vi "OutputLimeLight.vi"   [LabVIEW 2020]
doc: "This VI sends commands to the LimeLight camera."
uses:
  a4c4c9eb-852e-4134-b059-2c269de838ae.vi
  bed327a2-98d3-4965-916e-7305edcf582b.vi
  9959ab12-4f3e-4c63-8bb4-e3e2fa624083.vi
  a4c4c9eb-852e-4134-b059-2c269de838ae.vi/77c742ae-e671-49bb-a825-a6e8cebc9f63.vi
  bed327a2-98d3-4965-916e-7305edcf582b.vi/77c742ae-e671-49bb-a825-a6e8cebc9f63.vi
  9959ab12-4f3e-4c63-8bb4-e3e2fa624083.vi/77c742ae-e671-49bb-a825-a6e8cebc9f63.vi
  <vilib>/Rock Robotics/Network Tables/NT Read Number.vi
  GlobalMiscellaneous.vi
  GlobalDriverStationData.vi
  <vilib>/Rock Robotics/Network Tables/NT Write Value.vi
  <vilib>/Rock Robotics/Network Tables/NT Write Number.vi
types:
  T1 = enum16{"Side-by-Side", "PiP Main", "PiP Secondary"}
  T2 = enum16{"Boot Up", "Camera Override", "HUB Targeting", "CARGO Tracking"}
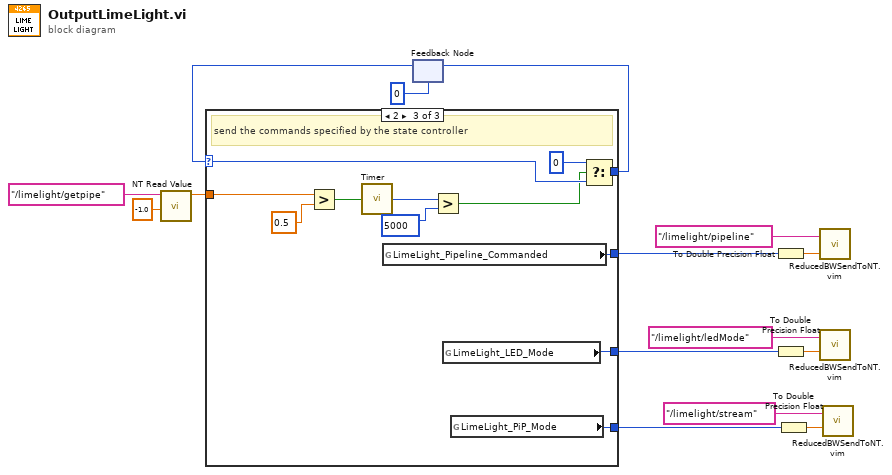
[diagram p0: block diagram]
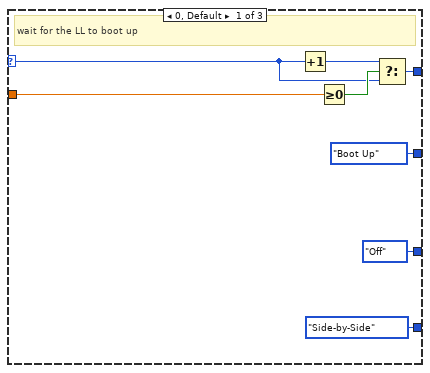
[diagram p2: hidden frame]
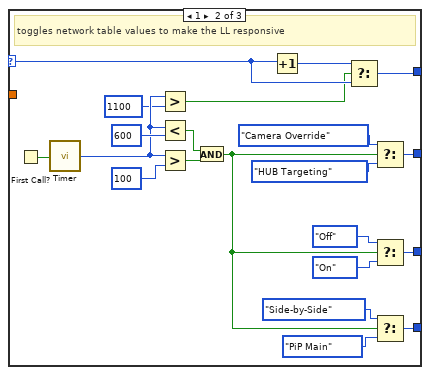
[diagram p3: hidden frame]
diagram:
  n1 = call-poly <vilib>:"NT Read Value.vi"("Default Value"=-1.0, "Name"="/limelight/getpipe") -> ("Numeric"=w6:dbl)  [unwired: 8 in, 1 out]
  n2 = feedback #1(0) -> (w10:i32)
  n3 = case shown="2" w10 {
    selector: w10 -> [w21 w43 w54]
    tunnel: [w20 w42 w55] -> w11
    tunnel: [T2."Boot Up" w28 w46] -> w5
    tunnel: [enum16{"Pipeline Setting", "Off", "Blink", "On"}."Off" ("LimeLight_LED_Mode") w29 w56] -> w4
    tunnel: w6 -> [w17 _ w52]
    tunnel: [T1."Side-by-Side" ("LimeLight_PiP_Mode") w27 w45] -> w1
    frame 0, Default {
      # "wait for the LL to boot up"
      n4 = Increment(x=w21) -> (x+1=w22:i32)
      n5 = Greater Or Equal To 0?(x=w17) -> (x >= 0?=w23:bool)
      n6 = Select(t=w22, s=w23, f=w21) -> (s? t:f=w20:i32)
    }
    frame 1 {
      # "toggles network table values to make the LL responsive"
      n7 = First Call?() -> (First Call?: T/F=w41:bool)
      n8 = call "Timer.vi"("Reset Timer"=w41) -> ("Time (ms)"=w34:u32)
      n9 = Greater?(x=w34, y=u32 1100) -> (0:w32:bool)
      n10 = Less?(x=w34, y=u32 600) -> (x < y?=w37:bool)
      n11 = Greater?(x=w34, y=u32 100) -> (0:w39:bool)
      n12 = And(x=w37, y=w39) -> (x .and. y?=w26:bool)
      n13 = Increment(x=w43) -> (x+1=w44:i32)
      n14 = Select(t=w44, s=w32, f=w43) -> (s? t:f=w42:i32)
      n15 = Select(t=T2."Camera Override", s=w26, f=T2."HUB Targeting") -> (s? t:f=w28:T2)
      n16 = Select(t=enum16{"Pipeline Setting", "Off", "Blink", "On"}."Off" ("LimeLight_LED_Mode"), s=w26, f=enum16{"Pipeline Setting", "Off", "Blink", "On"}."On" ("LimeLight_LED_Mode")) -> (s? t:f=w29:enum16{"Pipeline Setting", "Off", "Blink", "On"})
      n17 = Select(t=T1."Side-by-Side" ("LimeLight_PiP_Mode"), s=w26, f=T1."PiP Main") -> (s? t:f=w27:T1)
    }
    frame 2 {
      # "send the commands specified by the state controller"
      n18 = Greater?(x=w52, y=0.5 ("Numeric")) -> (0:w50:bool)
      n19 = call "Timer.vi"("Reset Timer"=w50) -> ("Time (ms)"=w49:u32)
      n20 = global read "GlobalMiscellaneous.vi" "LimeLight_Pipeline_Commanded"() -> (w46:T2)
      n21 = Greater?(x=w49, y=u32 5000) -> (0:w47:bool)
      n22 = global read "GlobalMiscellaneous.vi" "LimeLight_LED_Mode"() -> (w56:enum16{"Pipeline Setting", "Off", "Blink", "On"})
      n23 = global read "GlobalMiscellaneous.vi" "LimeLight_PiP_Mode"() -> (w45:T1)
      n24 = Select(t=0, s=w47, f=w54) -> (s? t:f=w55:i32)
    }
  }
  n25 = feedback-in #1(w11) -> ()
  n26 = To Double Precision Float(number=w5) -> (double precision float=w13:dbl)
  n27 = To Double Precision Float(number=w4) -> (double precision float=w15:dbl)
  n28 = To Double Precision Float(number=w1) -> (double precision float=w3:dbl)
  n29 = call "ReducedBWSendToNT.vim"("Value In"=w13, "NT Name"="/limelight/pipeline" ("Name")) -> ()  [unwired: 1 out]
  n30 = call "ReducedBWSendToNT.vim"("Value In"=w15, "NT Name"="/limelight/ledMode" ("Name")) -> ()  [unwired: 1 out]
  n31 = call "ReducedBWSendToNT.vim"("Value In"=w3, "NT Name"="/limelight/stream" ("Name")) -> ()  [unwired: 1 out]
